vi "AH_OpenFile.vi"(7 "Status Ref":refnum<vi>, 8 "error in":errorcluster, 10 "Config_Cluster":T1={"General"={"Config.ini"=path "", "Default Logging Path"=path ""}, "Hardware"={"AHC VISA COM"="", "Measure Rate (1/s)"=0, "Global T VAR"="", "Global B VAR"=""}, "Operation"={"Operation Mode"=enum."Idle-Off", "Status"="", "NewLog?"=FALSE}}) -> (0 "error out":errorcluster, 2 "Config_Cluster Out":T1={"General"={"Config.ini"=path "", "Default Logging Path"=path ""}, "Hardware"={"AHC VISA COM"="", "Measure Rate (1/s)"=0, "Global T VAR"="", "Global B VAR"=""}, "Operation"={"Operation Mode"=enum."Idle-Off", "Status"="", "NewLog?"=FALSE}}, 3 "refnum out":refnum<file>, 4 "FileOpen?":bool)   [LabVIEW 2021]
uses:
  Config_Cluster.ctl
  Mode_Enum.ctl
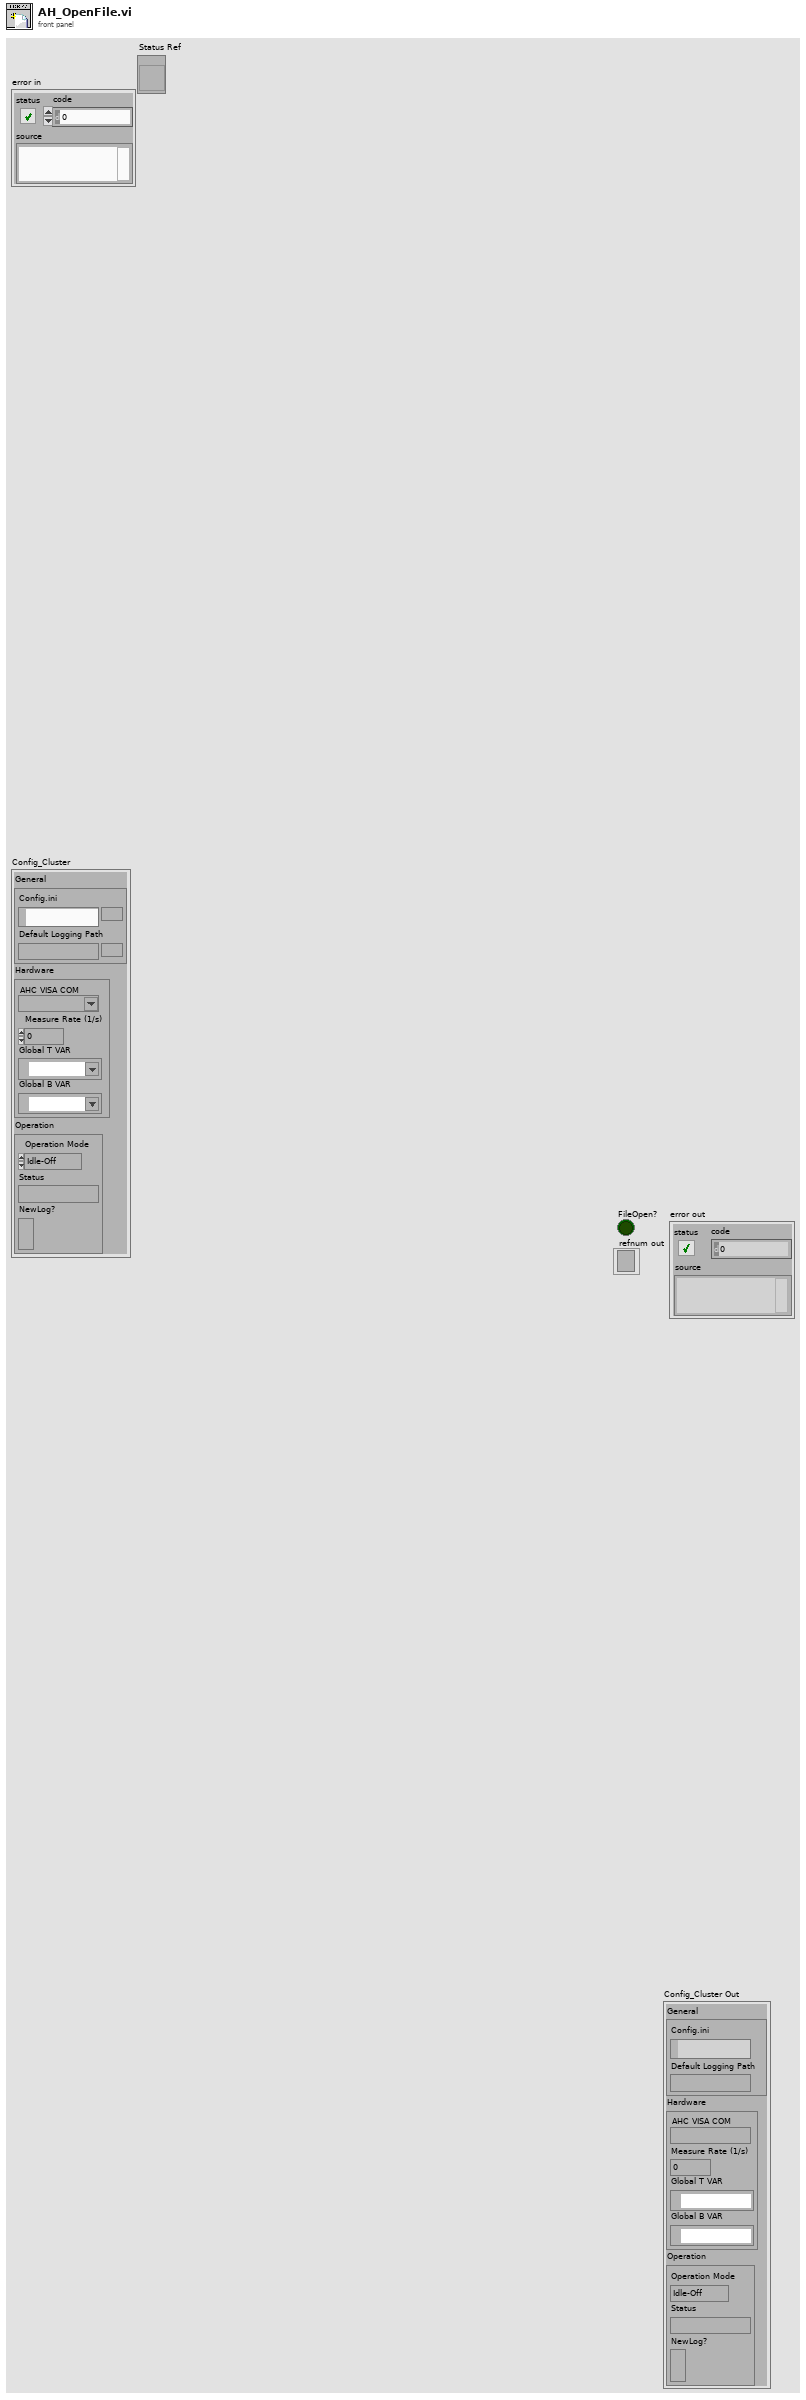
[diagram p1: front panel]
types:
  T1 = typedef "Config_Cluster.ctl" = cluster{"General":cluster{"Config.ini":path, "Default Logging Path":path}, "Hardware":cluster{"AHC VISA COM":refnum<visa-resource-name>, "Measure Rate (1/s)":i32, "Global T VAR":refnum<k21>, "Global B VAR":refnum<k21>}, "Operation":cluster{"Operation Mode":T2, "Status":string, "NewLog?":bool}}
  T2 = typedef "Mode_Enum.ctl" = enum16{"Logging", "Idle-Off", "Idle"}
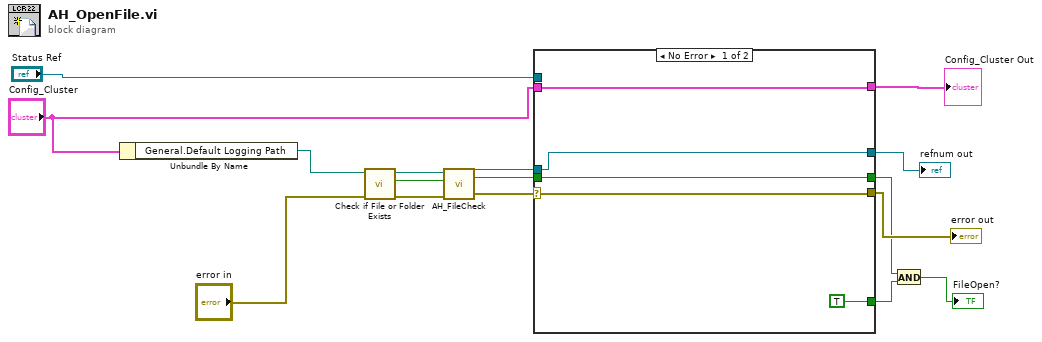
[diagram p0: block diagram]
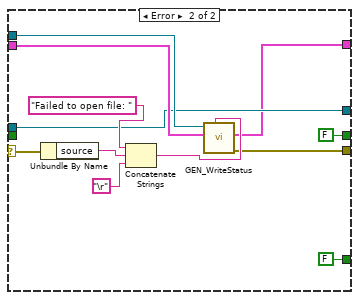
[diagram p2: hidden frame]
diagram:
  n1 = Unbundle By Name("Config_Cluster") -> ("General.Default Logging Path"=w13:path)
  n2 = call <vilib>:"Check if File or Folder Exists.vi"("error in (no error)"="error in", "path"=w13) -> ("error out"=w7:errorcluster, "file or folder exists?"=w8:bool, "dup path"=w9:path)  [unwired: 7 in]
  n3 = call "AH_FileCheck.vi"("error in"=w7, "Exists"=w8, "Path IN"=w9) -> ("error Out"=w4:errorcluster, "Continue"=w5:bool, "refnum"=w6:refnum<file>)  [unwired: 6 in]
  n4 = case shown="No Error" w4 {
    selector: w4 -> [w21 w31]
    tunnel: w6 -> [w20 w25]
    tunnel: "Status Ref" -> [_ w33]
    tunnel: "Config_Cluster" -> [w18 w32]
    tunnel: [w21 w26] -> w11
    tunnel: [w20 w25] -> w12
    tunnel: [TRUE FALSE] -> w2
    tunnel: [w18 w23] -> w10
    tunnel: w5 -> [w17 _]
    tunnel: [w17 FALSE ("Continue")] -> w1
    frame No Error {
    }
    frame Error {
      n5 = Unbundle By Name(w31) -> ("source"=w29:string)
      n6 = Concatenate Strings("Failed to open file: " ("string"), w29, "\r") -> (w27:string)
      n7 = call "GEN_WriteStatus.vi"("Input String"=w27, "Config_Cluster"=w32, "Status Ref"=w33) -> ("error out"=w26:errorcluster, "Config_Cluster Out"=w23:T1)  [unwired: 7 in]
    }
  }
  "refnum out" <- w12
  "error out" <- w11
  "Config_Cluster Out" <- w10
  n8 = And(x=w1, y=w2) -> (x .and. y?=→"FileOpen?":bool)
